vi "to_json.vi"(8 "error in":errorcluster, 11 "scaleFactor in":refnum<class "scaleFactor.lvclass">) -> (0 "error out":errorcluster, 2 "json":string, 3 "scaleFactor out":refnum<class "scaleFactor.lvclass">, 4 "Not Default":bool)   [LabVIEW 2020, in "nominal types.lvlib" / "timestampManifest.lvlib" / "scaleFactor.lvclass"]
uses:
  scaleFactor.lvclass
  scaleFactor.lvclass/scaleFactor.ctl
  9065bcfc-cb62-4650-b7ab-74173ce26db5.vi
  <vilib>/JDP Science/JSONtext/Variant to JSON Text.vi
  <vilib>/JDP Science/JSONtext/LVClass Serializer/JSONtext LVClass Serializer.lvclass
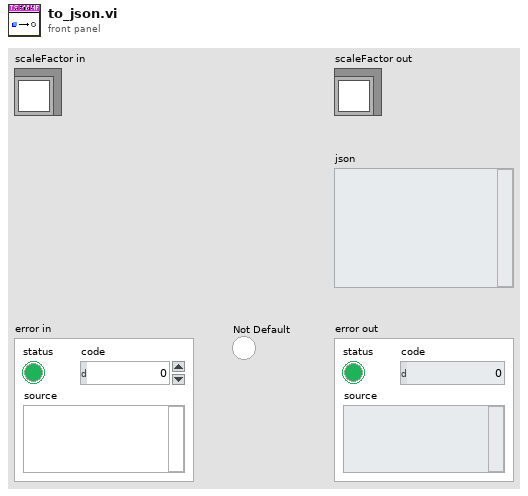
[diagram p1: front panel]
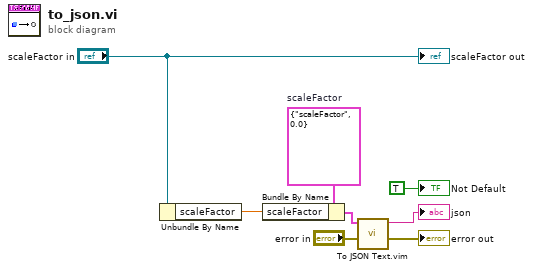
[diagram p0: block diagram]
diagram:
  w6 = cluster{"type":string, "scaleFactor":dbl} {"type"="scaleFactor", "scaleFactor"=0.0}  # scaleFactor
  n1 = Unbundle By Name("scaleFactor in") -> ("scaleFactor"=w7:dbl)
  n2 = Bundle By Name(cluster=w6, "scaleFactor"=w7) -> (w5:cluster{"type":string, "scaleFactor":dbl})
  n3 = call "To JSON Text.vim"("error in (no error)"="error in", "Anything"=w5) -> ("error out"=→"error out":errorcluster, "<JSON>"=→"json":string)  [unwired: 8 in]
  "scaleFactor out" <- "scaleFactor in"
  "Not Default" <- TRUE ("Not Default")
